vi "PID_model_01.vi"() -> ()   [LabVIEW 2022 SP3]
uses:
  <vilib>/Platform/TimedLoop/XDataNode/timing_clust.ctl
  <vilib>/Platform/TimedLoop/XDataNode/nitl_modes.ctl
  <vilib>/Platform/TimedLoop/XDataNode/wakeup.ctl
  <vilib>/Utility/file.llb/Read Delimited Spreadsheet (DBL).vi
  <vilib>/Platform/TimedLoop/scheduler/LVUserAPI/_suppVIs/Create_1kHz_TSource.vi
  <vilib>/platform/TimedLoop/XDataNode/XDataNode.xnode
  <vilib>/Platform/TimedLoop/XDataNode/XDNodeRunTimeDep.lvlib
  <vilib>/addons/control/pid/NI_PID_pid.lvlib
  <vilib>/gmath/NI_Gmath.lvlib
  <vilib>/addons/control/pid/pid.llb/PID (DBL).vi
  <vilib>/measure/NI_MABase.lvlib
panel:
  in  "method":i32(ring)=1 items=["nearest", "linear", "spline", "cubic Hermite", "Lagrange"]
  in  "stop":bool
  in  "Excitation Source":T1(tab)
  in  "Cluster":T2={"frequency"=3.0, "amplitude"=1.0, "signal type"=enum."Sine Wave"} {"amplitude" format="%0.2p"; "frequency" format="%0.2p"}
  in  "Cluster 2":cluster{"standard deviation":dbl}={"standard deviation"=1.0} {"standard deviation" format="%.2p"}
  out "Plant Output":dbl[](graph)
  in  "Proportional Gain":dbl
  in  "Setpoint":dbl
  in  "cluster":T3={"Initial X Axis Value"=0, "X Axis Increment"=6.10352, []}
  out "Excitation & Response FRFs":T4(graph)
  out "Phase 2":cluster{"Array":dbl[], "Array":dbl[]}(graph) caption="Amplitude [Hz]"
  in  "Skip First N Lines 2":i32=48
  out "Magnitude 2":cluster{"Array":dbl[], "Array":dbl[]}(graph) caption="Amplitude [Hz]"
  out "number of rows 2":i32
  in  "name or relative path 2":path=path "C:/Users/LAV-UFSC/OneDrive - UFSC/Documents/LAV - TCC/Dados-Experimentos/25-04/frf_8.txt"
  out "Phase":cluster{"Array":dbl[], "Array":dbl[]}(graph) caption="Amplitude [Hz]"
  in  "Skip First N Lines":i32=48
  out "Magnitude":cluster{"Array":dbl[], "Array":dbl[]}(graph) caption="Amplitude [Hz]"
  out "number of rows":i32
  in  "name or relative path":path=path "C:/Users/LAV-UFSC/OneDrive - UFSC/Documents/LAV - TCC/Dados-Experimentos/25-04/frf_3.txt"
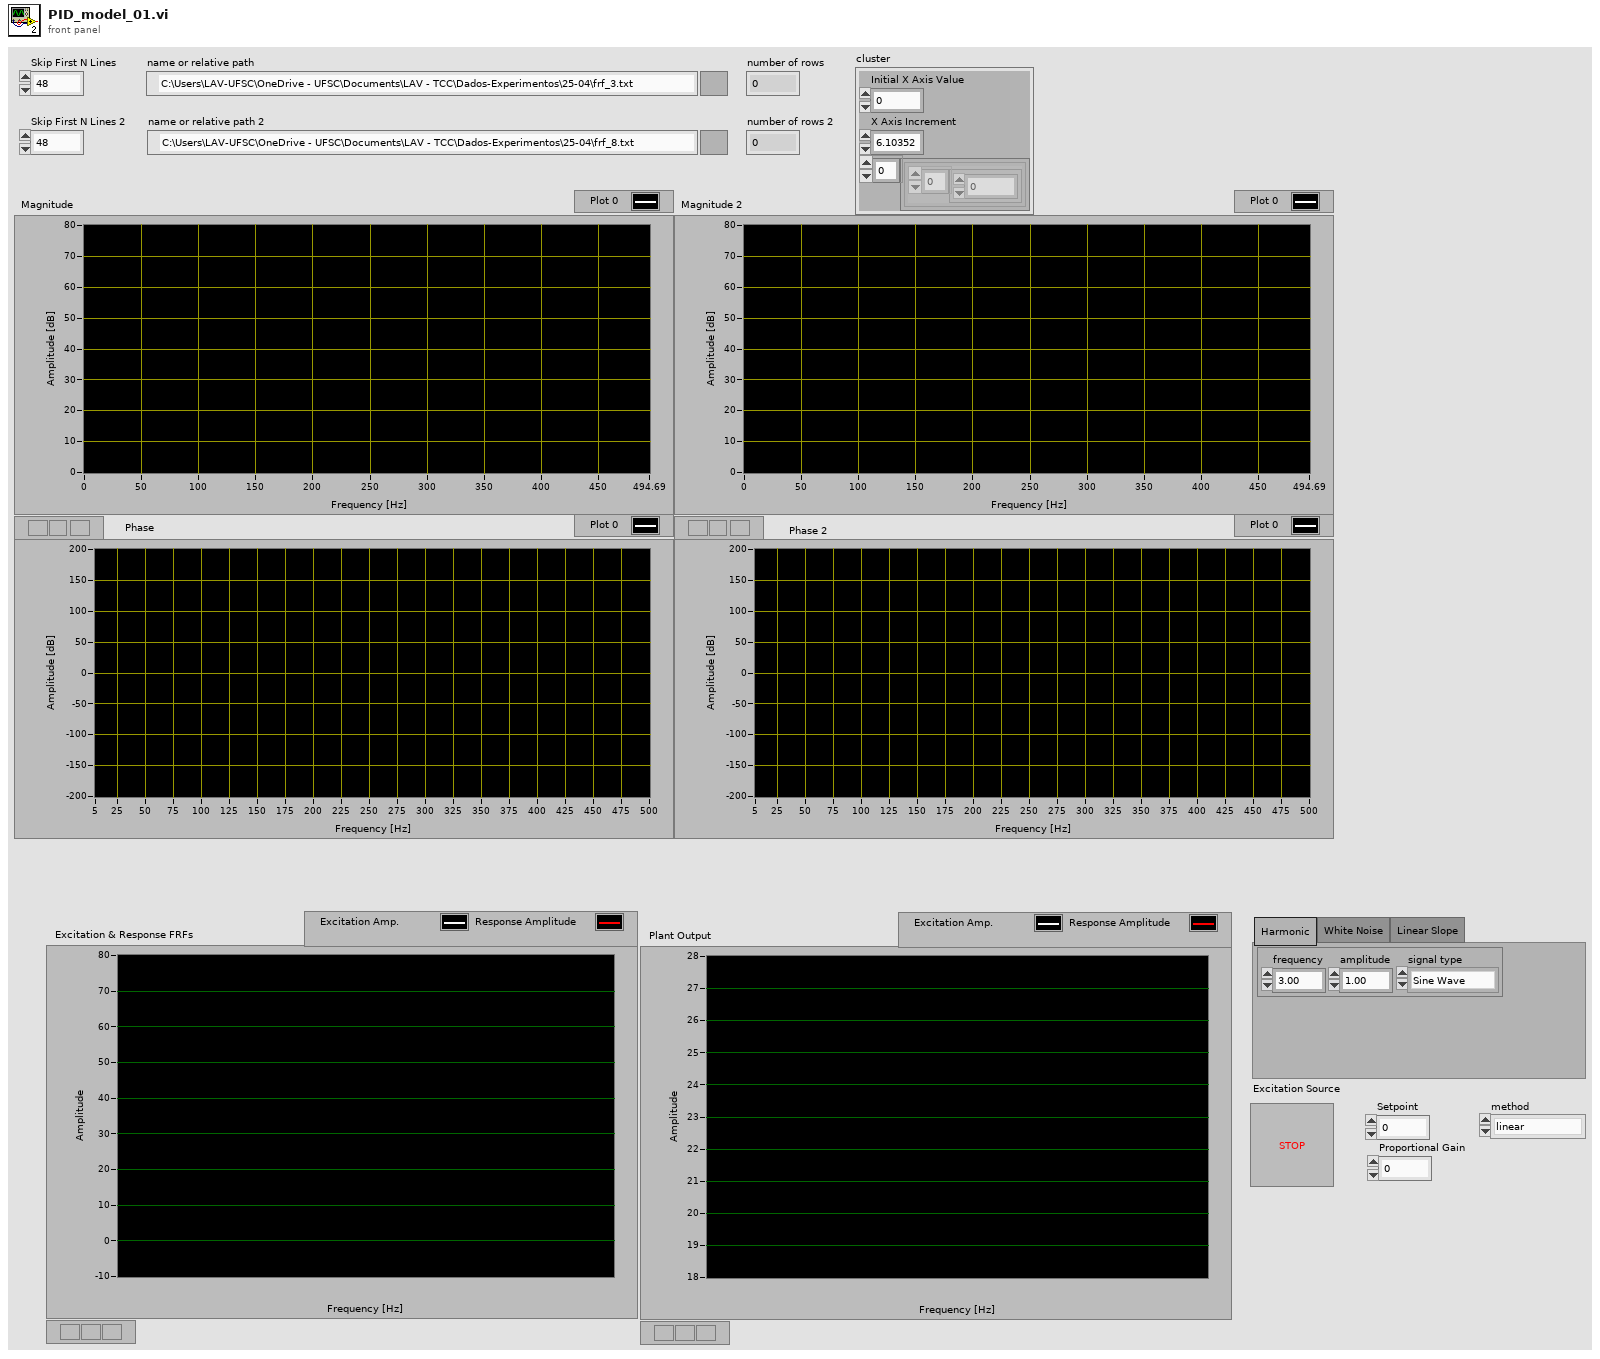
[diagram p1: front panel]
types:
  T1 = enum32{"Harmonic", "White Noise", "Linear Slope"}
  T2 = cluster{"frequency":dbl, "amplitude":dbl, "signal type":enum16{"Sine Wave", "Triangle Wave", "Square Wave", "Sawtooth Wave"}}
  T3 = cluster{"Initial X Axis Value":i32, "X Axis Increment":dbl, cluster{dbl[]}[]}
  T4 = cluster{i32, "X Axis Increment":dbl, cluster{dbl[]}[]}
  T5 = typedef "XDNodeRunTimeDep.lvlib/timing_clust.ctl" = cluster{"Expected End [f-1]":u64, "Actual End [f-1]":u64, "Finished Late? [f-1]":bool, "Expected End [i-1]":u64, "Actual End [i-1]":u64, "Finished Late? [i-1]":bool, "Expected Start [i]":u64, "Actual Start [i]":u64, "Expected Start [f]":u64, "Actual Start [f]":u64, "Source Name":string, "Structure Name":string, "Period":i64, "Deadline":i64, "Offset":i64, "Start":i64, "Priority":i32, "Timeout":i32, "Mode":T6, "Wakeup Reason":T7, "Error":errorcluster, "Source Type":string, "Secondary Source Type":string, "Global End Time":u64, "Global Start Time":u64, "Frame Duration":u64, "Iteration Duration":u64, "Assigned CPU":i32, "I/O Scan Engine Mode":u32}
  T6 = typedef "XDNodeRunTimeDep.lvlib/nitl_modes.ctl" = enum32{"No Change", "Process missed periods, maintain original phase", "Discard missed periods, maintain original phase", "Process missed periods, ignore original phase", "Discard missed periods, ignore original phase"}
  T7 = typedef "XDNodeRunTimeDep.lvlib/wakeup.ctl" = enum32{"Normal", "Aborted", "Asynchronous wakeup", "Timing source error", "Timed loop error", "Timeout"}
  T8 = enum16{"Sine Wave", "Triangle Wave", "Square Wave", "Sawtooth Wave"}
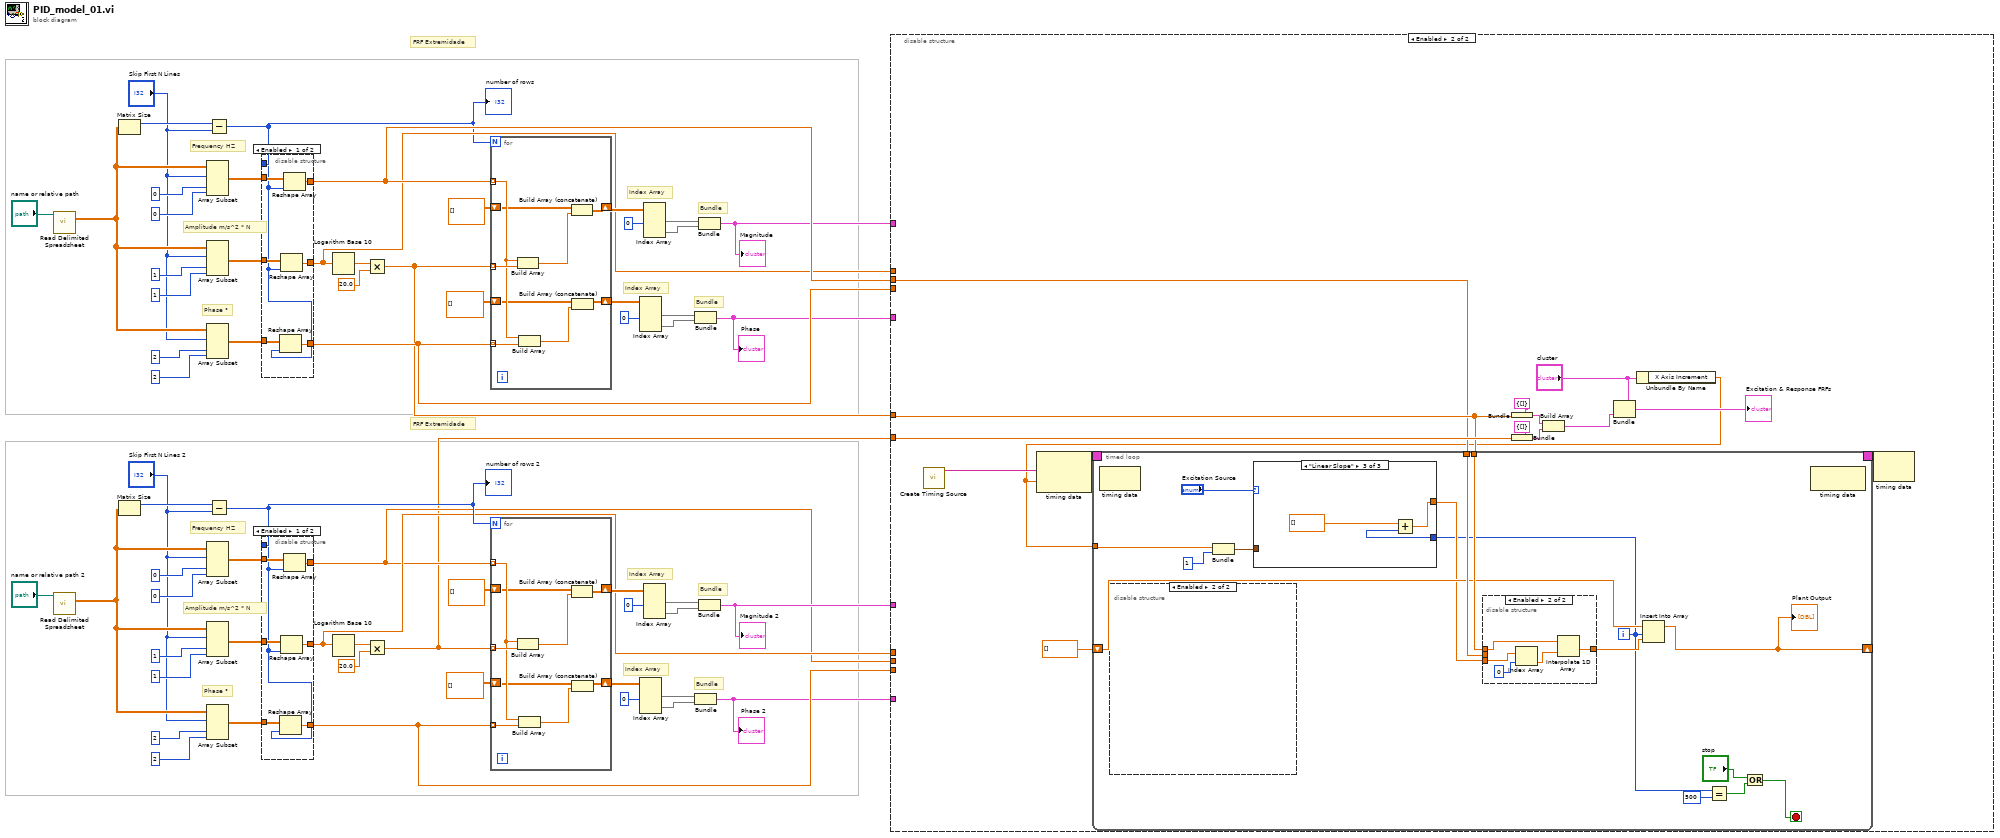
[diagram p0: block diagram]
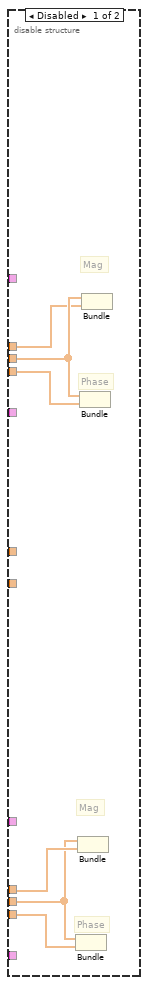
[diagram p3: hidden frame]
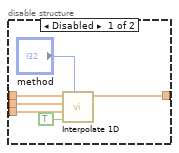
[diagram p4: hidden frame]
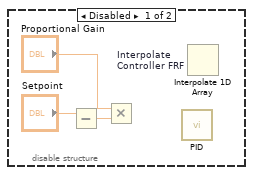
[diagram p5: hidden frame]
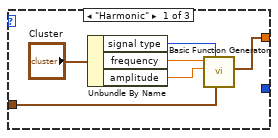
[diagram p6: hidden frame]
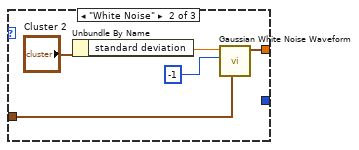
[diagram p7: hidden frame]
diagram:
  # "FRF Extremidade"
  # "Index Array"
  # "Bundle"
  # "Index Array"
  # "Bundle"
  # "Phase °"
  # "Amplitude m/s^2 * N"
  # "Frequency HZ"
  # "FRF Extremidade"
  # "Index Array"
  # "Bundle"
  # "Index Array"
  # "Bundle"
  # "Phase °"
  # "Amplitude m/s^2 * N"
  # "Frequency HZ"
  n1 = call-poly <vilib>:"Read Delimited Spreadsheet.vi"("file path (dialog if empty)"="name or relative path") -> ("all rows"=w55:dbl[][])  [unwired: 9 in, 5 out]
  n2 = call-poly <vilib>:"Read Delimited Spreadsheet.vi"("file path (dialog if empty)"="name or relative path 2") -> ("all rows"=w24:dbl[][])  [unwired: 9 in, 5 out]
  n3 = Matrix Size(0:w55) -> (1:w38:i32)  [unwired: 1 out]
  n4 = Matrix Size(0:w24) -> (1:w10:i32)  [unwired: 1 out]
  n5 = Array Subset(array=w55, index (row)="Skip First N Lines", index (col)=0 ("column 1"), length (col)=0 ("column N")) -> (w57:dbl[][])  [unwired: 1 in]
  n6 = Array Subset(array=w55, index (row)="Skip First N Lines", index (col)=1 ("column 1"), length (col)=1 ("column N")) -> (w56:dbl[][])  [unwired: 1 in]
  n7 = Array Subset(array=w55, index (row)="Skip First N Lines", index (col)=2 ("column 1"), length (col)=2 ("column N")) -> (w40:dbl[][])  [unwired: 1 in]
  n8 = Array Subset(array=w24, index (row)="Skip First N Lines 2", index (col)=0 ("column 1"), length (col)=0 ("column N")) -> (w26:dbl[][])  [unwired: 1 in]
  n9 = Array Subset(array=w24, index (row)="Skip First N Lines 2", index (col)=1 ("column 1"), length (col)=1 ("column N")) -> (w25:dbl[][])  [unwired: 1 in]
  n10 = Array Subset(array=w24, index (row)="Skip First N Lines 2", index (col)=2 ("column 1"), length (col)=2 ("column N")) -> (w11:dbl[][])  [unwired: 1 in]
  n11 = Subtract(x=w38, y="Skip First N Lines") -> (x-y=w36:i32)
  "number of rows" <- w36
  n12 = Subtract(x=w10, y="Skip First N Lines 2") -> (x-y=w8:i32)
  "number of rows 2" <- w8
  n13 = disable-structure shown="Enabled" {
    disable-tunnel: w57 -> [w71 w73]
    disable-tunnel: w56 -> [w70 w72]
    disable-tunnel: [w69 w73] -> w42
    disable-tunnel: [w68 w72] -> w41
    disable-tunnel: w36 -> [w66 _]
    disable-tunnel: w40 -> [w67 _]
    disable-tunnel: [w65 _] -> w39
    frame Enabled {
      n14 = Reshape Array(w67, w66) -> (w65:dbl[])
      n15 = Reshape Array(w70, w66) -> (w68:dbl[])
      n16 = Reshape Array(w71, w66) -> (w69:dbl[])
    }
    frame Disabled {
    }
  }
  n17 = disable-structure shown="Enabled" {
    disable-tunnel: w26 -> [w80 w82]
    disable-tunnel: w25 -> [w79 w81]
    disable-tunnel: [w78 w82] -> w5
    disable-tunnel: [w77 w81] -> w6
    disable-tunnel: w8 -> [w75 _]
    disable-tunnel: w11 -> [w76 _]
    disable-tunnel: [w74 _] -> w4
    frame Enabled {
      n18 = Reshape Array(w76, w75) -> (w74:dbl[])
      n19 = Reshape Array(w79, w75) -> (w77:dbl[])
      n20 = Reshape Array(w80, w75) -> (w78:dbl[])
    }
    frame Disabled {
    }
  }
  n21 = Logarithm Base 10(1:w41) -> (0:w48:dbl[])
  n22 = Logarithm Base 10(1:w6) -> (0:w17:dbl[])
  n23 = Multiply(x=w48, y=20.0) -> (x*y=w1:dbl[])
  n24 = Multiply(x=w17, y=20.0) -> (x*y=w2:dbl[])
  n25 = for {
    N: w36 -> [_]
    tunnel: w42 -> [w89] mode=indexing
    tunnel: w1 -> [w90] mode=indexing
    tunnel: w39 -> [w91] mode=indexing
    shift-right: [w86] -> w50
    shift-left: dbl[][] [] -> [w88]
    shift-right: [w85] -> w43
    shift-left: dbl[][] [] -> [w84]
    n26 = Build Array(w89, w90) -> (w87:dbl[])
    n27 = Build Array(w89, w91) -> (w83:dbl[])
    n28 = Build Array (concatenate)(w88, w87) -> (w86:dbl[][])
    n29 = Build Array (concatenate)(w84, w83) -> (w85:dbl[][])
  }
  n30 = for {
    N: w8 -> [_]
    tunnel: w5 -> [w98] mode=indexing
    tunnel: w2 -> [w99] mode=indexing
    tunnel: w4 -> [w100] mode=indexing
    shift-right: [w95] -> w19
    shift-left: dbl[][] [] -> [w97]
    shift-right: [w94] -> w12
    shift-left: dbl[][] [] -> [w93]
    n31 = Build Array(w98, w99) -> (w96:dbl[])
    n32 = Build Array(w98, w100) -> (w92:dbl[])
    n33 = Build Array (concatenate)(w97, w96) -> (w95:dbl[][])
    n34 = Build Array (concatenate)(w93, w92) -> (w94:dbl[][])
  }
  n35 = Index Array(array=w43, index (col) #1=0 ("disabled index (col)")) -> (element #1=w44:dbl[], element #2=w45:dbl[])  [unwired: 3 in]
  n36 = Index Array(array=w12, index (col) #1=0 ("disabled index (col)")) -> (element #1=w13:dbl[], element #2=w14:dbl[])  [unwired: 3 in]
  n37 = Index Array(array=w50, index (col) #1=0 ("disabled index (col)")) -> (element #1=w51:dbl[], element #2=w52:dbl[])  [unwired: 3 in]
  n38 = Index Array(array=w19, index (col) #1=0 ("disabled index (col)")) -> (element #1=w20:dbl[], element #2=w21:dbl[])  [unwired: 3 in]
  n39 = Bundle(w44, w45) -> (w34:cluster{dbl[], dbl[]})  [unwired: 1 in]
  "Phase" <- w34
  n40 = Bundle(w13, w14) -> (w3:cluster{dbl[], dbl[]})  [unwired: 1 in]
  "Phase 2" <- w3
  n41 = Bundle(w51, w52) -> (w35:cluster{dbl[], dbl[]})  [unwired: 1 in]
  "Magnitude" <- w35
  n42 = Bundle(w20, w21) -> (w7:cluster{dbl[], dbl[]})  [unwired: 1 in]
  "Magnitude 2" <- w7
  n43 = disable-structure shown="Enabled" {
    disable-tunnel: w42 -> [w106 w111]
    disable-tunnel: w41 -> [w105 _]
    disable-tunnel: w39 -> [w104 _]
    disable-tunnel: w35 -> [_ _]
    disable-tunnel: w34 -> [_ _]
    disable-tunnel: w7 -> [_ _]
    disable-tunnel: w6 -> [w103 _]
    disable-tunnel: w5 -> [w101 _]
    disable-tunnel: w4 -> [w102 _]
    disable-tunnel: w3 -> [_ _]
    disable-tunnel: w2 -> [_ w117]
    disable-tunnel: w1 -> [_ w114]
    frame Disabled {
      # "Phase"
      # "Mag"
      # "Phase"
      # "Mag"
      n44 = Bundle("all rows"=w101, "all rows"=w102) -> ()  [unwired: 2 out]
      n45 = Bundle("all rows"=w101, "all rows"=w103) -> ()  [unwired: 2 out]
      n46 = Bundle("all rows"=w106, "all rows"=w104) -> ()  [unwired: 2 out]
      n47 = Bundle("all rows"=w106, "all rows"=w105) -> ()  [unwired: 2 out]
    }
    frame Enabled {
      n48 = call-poly <vilib>:"Create Timing Source.vi"() -> ("name (out)"=w109:string)  [unwired: 10 in, 1 out]
      n49 = Bundle(cluster=cluster{dbl[]} {[]} ("Excitation Amplitude [dB]"), w114) -> (w121:cluster{dbl[]})
      n50 = Bundle(cluster=cluster{dbl[]} {[]} ("Response Amplitude [dB]"), w117) -> (w120:cluster{dbl[]})
      n51 = Build Array(w121, w120) -> (w119:cluster{dbl[]}[])
      n52 = Bundle(cluster="cluster", w119) -> (→"Excitation & Response FRFs":T3)  [unwired: 2 in]
      n53 = Unbundle By Name("cluster") -> ("X Axis Increment"=w108:dbl)
      n54 = node-c288(w109, w108) -> (w113:T5)
      n55 = timed-loop {
        tunnel: w114 -> [w135]
        timing: w113 -> [_]
        timing-out: [_] -> w112
        tunnel: w111 -> [w134]
        shift-right: [w128] -> _
        shift-left: dbl[] [] ("yi") -> [w133]
        tunnel: w108 -> [w131]
        i -> [w123]
        stop <- w125 stop-if-true
        n56 = node-c288() -> ()  [unwired: 1 in, 1 out]
        n57 = disable-structure shown="Enabled" {
          frame Disabled {
            n58 = Subtract(x="Setpoint") -> (y=w148:dbl, x-y=w150:dbl)
            n59 = Multiply(x="Proportional Gain", y=w150) -> ()  [unwired: 1 out]
            n60 = call-poly <vilib>:"PID.vi"() -> ()  [unwired: 10 in, 2 out]
            n61 = Interpolate 1D Array "Interpolate\nController FRF"() -> ()  [unwired: 2 in, 1 out]
          }
          frame Enabled {
          }
        }
        n62 = Bundle("X Axis Increment"=w131, 1) -> (w130:cluster{"X Axis Increment":dbl, i32})  [unwired: 1 in]
        n63 = case shown="\"Linear Slope\"" "Excitation Source" {
          tunnel: w130 -> [w153 w159 _]
          tunnel: [w152 w158 w165] -> w129
          tunnel: w123 -> [_ _ w163]
          frame "Harmonic" {
            n64 = Unbundle By Name("Cluster") -> ("signal type"=w154:T8, "frequency"=w155:dbl, "amplitude"=w156:dbl)
            n65 = call <vilib>:"Basic Function Generator.vi"("sampling info"=w153, "signal type"=w154, "amplitude"=w156, "frequency"=w155) -> ("signal out"=w152:waveform(dbl))  [unwired: 5 in, 2 out]
          }
          frame "White Noise" {
            n66 = Unbundle By Name("Cluster 2") -> ("standard deviation"=w161:dbl)
            n67 = call <vilib>:"Gaussian White Noise Waveform.vi"("sampling info"=w159, "seed"=-1, "standard deviation"=w161) -> ("signal out"=w158:waveform(dbl))  [unwired: 7 in, 1 out]
          }
          frame "Linear Slope" {
            n68 = Add(x=dbl[] [] ("xi"), y=w163) -> (x+y=w165:dbl[])
          }
        }
        n69 = disable-structure shown="Enabled" {
          disable-tunnel: w135 -> [w142 w146]
          disable-tunnel: w134 -> [w141 _]
          disable-tunnel: w129 -> [w139 w145]
          disable-tunnel: [w138 w147] -> w127
          frame Disabled {
            n70 = call <vilib>:"Interpolate 1D.vi"("method"="method", "X is monotonic"=TRUE, "xi"=w139, "X"=w141, "Y"=w142) -> ("yi"=w138:dbl[])  [unwired: 4 in, 2 out]
          }
          frame Enabled {
            n71 = Index Array(array=w145, index=0) -> (element=w143:dbl)
            n72 = Interpolate 1D Array(1:w143, 2:w146) -> (0:w147:dbl)
          }
        }
        n73 = Insert Into Array(array=w133, index=w123, new element=w127) -> (w128:dbl[])
        "Plant Output" <- w128
        n74 = Equal?(x=w123, y=500) -> (x = y?=w124:bool)
        n75 = Or(x="stop", y=w124) -> (x .or. y?=w125:bool)
        n76 = node-c288() -> ()  [unwired: 1 in, 1 out]
      }
      n77 = node-c288(w112) -> ()  [unwired: 1 out]
    }
  }
